vi "FP calculate steering angle.vi"(1 "Compass\nheading":dbl format="%#_13g", 2 "New heading":dbl format="%#_13g", 3 "Speed":i32) -> (0 "Local Steering Angle":dbl)   [LabVIEW 2014]
doc: "This VI calculates a steering angle in the local coordinates based upon the present compass heading and a desired new heading."
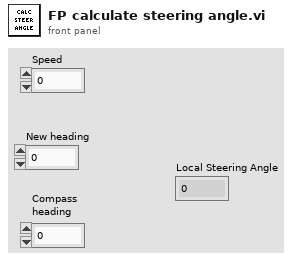
[diagram p1: front panel]
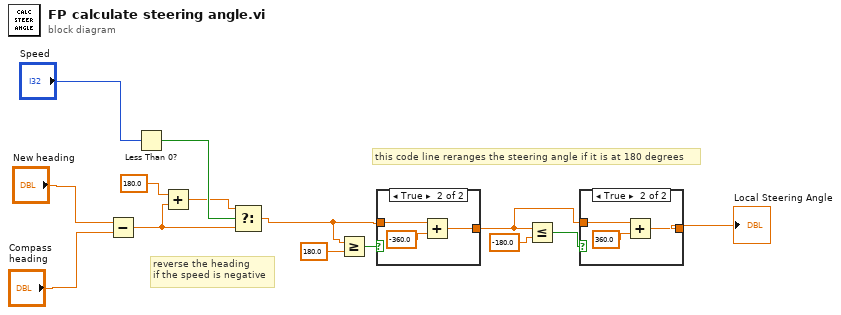
[diagram p0: block diagram]
diagram:
  # "reverse the heading\nif the speed is negative"
  # "this code line reranges the steering angle if it is at 180 degrees"
  n1 = Subtract(x="New heading", y="Compass\nheading") -> (x-y=w2:dbl)
  n2 = Less Than 0?(x="Speed") -> (x < 0?=w5:bool)
  n3 = Add(x=180.0, y=w2) -> (x+y=w3:dbl)
  n4 = Select(t=w3, s=w5, f=w2) -> (s? t:f=w1:dbl)
  n5 = Greater Or Equal?(x=w1, y=180.0) -> (x >= y?=w9:bool)
  n6 = case shown="True" w9 {
    tunnel: w1 -> [w15 w18]
    tunnel: [w15 w16] -> w6
    frame False {
    }
    frame True {
      n7 = Add(x=w18, y=-360.0) -> (x+y=w16:dbl)
    }
  }
  n8 = Less Or Equal?(x=w6, y=-180.0) -> (x <= y?=w7:bool)
  n9 = case shown="True" w7 {
    tunnel: w6 -> [w19 w22]
    tunnel: [w19 w20] -> w12
    frame False {
    }
    frame True {
      n10 = Add(x=w22, y=360.0) -> (x+y=w20:dbl)
    }
  }
  "Local Steering Angle" <- w12
